vi "量測_IO.vi"(7 "IO_Action":T2(ring), 8 "Error in":errorcluster, 11 "IO In":T1 {"Port" items=["Input Port #1", "Input Port #2", "Out Port #1", "Out Port #2"]}) -> (0 "Error Out":errorcluster, 3 "IO Out":T1 {"Port" items=["Input Port #1", "Input Port #2", "Out Port #1", "Out Port #2"]})   [LabVIEW 2015]
uses:
  Control/Main_IO #.ctl
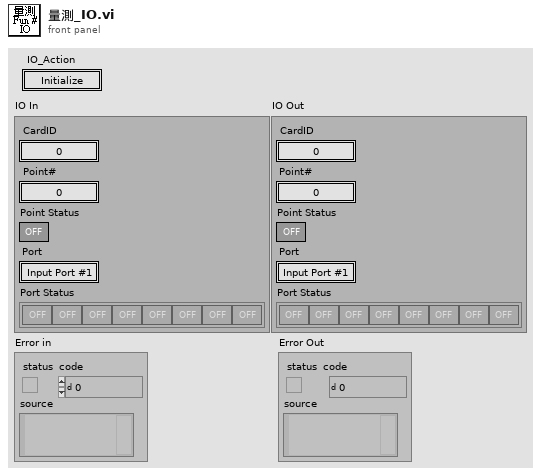
[diagram p1: front panel]
types:
  T1 = typedef "Main_IO #.ctl" = cluster{"CardID":u8, "Point#":u8, "Point Status":bool, "Port":u8, "Port Status":bool[]}
  T2 = enum16{"Initialize", "Set Point", "Set Port", "Read Point", "Read Port", "Close", "Idle"}
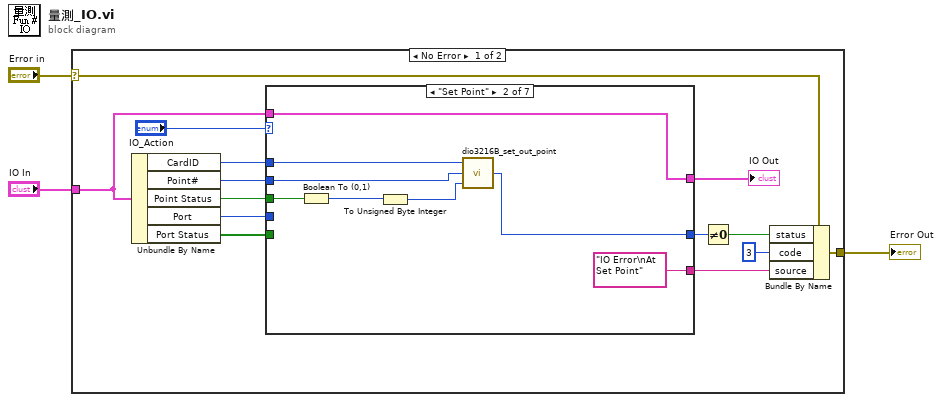
[diagram p0: block diagram]
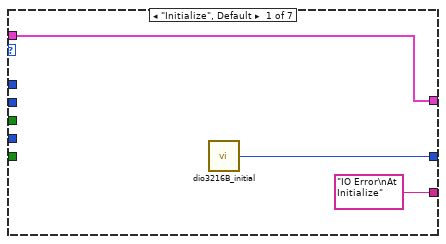
[diagram p2: hidden frame]
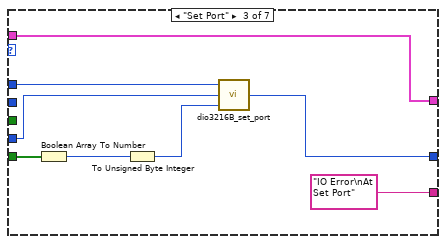
[diagram p3: hidden frame]
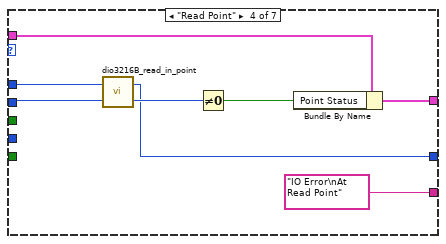
[diagram p4: hidden frame]
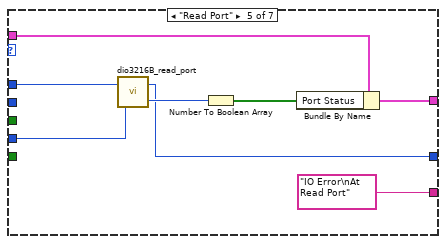
[diagram p5: hidden frame]
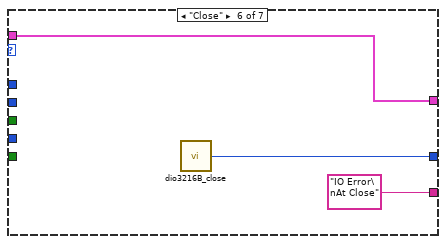
[diagram p6: hidden frame]
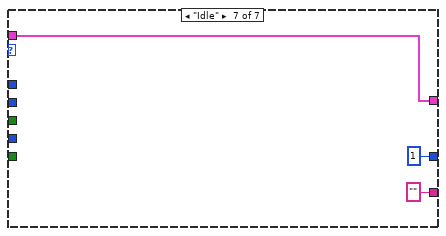
[diagram p7: hidden frame]
diagram:
  n1 = case shown="No Error" "Error in" {
    selector: "Error in" -> [w6 w59]
    tunnel: "IO In" -> [w12 _]
    tunnel: [w10 w59] -> w2
    frame No Error {
      n2 = Unbundle By Name(w12) -> ("CardID"=w17:u8, "Point#"=w16:u8, "Point Status"=w14:bool, "Port"=w15:u8, "Port Status"=w13:bool[])
      n3 = case shown="\"Set Point\"" "IO_Action" {
        tunnel: w17 -> [_ w28 w36 w44 w52 _ _]
        tunnel: w16 -> [_ w27 _ w43 _ _ _]
        tunnel: w14 -> [_ w26 _ _ _ _ _]
        tunnel: w15 -> [_ _ w35 _ w51 _ _]
        tunnel: w13 -> [_ _ w34 _ _ _ _]
        tunnel: w12 -> [w20 w23 w31 w42 w48 w55 w58]
        tunnel: [w20 w23 w31 w41 w49 w55 w58] -> w5
        tunnel: [w19 w22 w30 w38 w46 w54 u32 1 ("error_code")] -> w11
        tunnel: ["IO Error\nAt Initialize" "IO Error\nAt Set Point" "IO Error\nAt Set Port" "IO Error\nAt Read Point" "IO Error\nAt Read Port" "IO Error\nAt Close" ""] -> w7
        frame "Initialize", Default {
          n4 = call "dio3216B_initial.vi"() -> ("error_code"=w19:u32)
        }
        frame "Set Point" {
          n5 = Boolean To (0,1)(Boolean=w26) -> (0, 1=w25:i16)
          n6 = To Unsigned Byte Integer(number=w25) -> (unsigned 8bit integer=w24:u8)
          n7 = call "dio3216B_set_out_point.vi"("state"=w24, "point"=w27, "CardID"=w28) -> ("error_code"=w22:u32)
        }
        frame "Set Port" {
          n8 = Boolean Array To Number(Boolean array=w34) -> (number=w33:u32)
          n9 = To Unsigned Byte Integer(number=w33) -> (unsigned 8bit integer=w32:u8)
          n10 = call "dio3216B_set_port.vi"("data"=w32, "port"=w35, "CardID"=w36) -> ("error_code"=w30:u32)
        }
        frame "Read Point" {
          n11 = call "dio3216B_read_in_point.vi"("point"=w43, "CardID"=w44) -> ("state"=w40:u8, "error_code"=w38:u32)
          n12 = Not Equal To 0?(x=w40) -> (x != 0?=w39:bool)
          n13 = Bundle By Name(cluster=w42, "Point Status"=w39) -> (w41:T1)
        }
        frame "Read Port" {
          n14 = call "dio3216B_read_port.vi"("port"=w51, "CardID"=w52) -> ("data"=w50:u8, "error_code"=w46:u32)
          n15 = Number To Boolean Array(number=w50) -> (Boolean array=w47:bool[])
          n16 = Bundle By Name(cluster=w48, "Port Status"=w47) -> (w49:T1)
        }
        frame "Close" {
          n17 = call "dio3216B_close.vi"() -> ("error_code"=w54:u32)
        }
        frame "Idle" {
        }
      }
      "IO Out" <- w5
      n18 = Not Equal To 0?(x=w11) -> (x != 0?=w9:bool)
      n19 = Bundle By Name(cluster=w6, "status"=w9, "code"=3, "source"=w7) -> (w10:errorcluster)
    }
    frame Error {
    }
  }
  "Error Out" <- w2
